vi "_IgnoreInternalData.vi"(8 "error in (no error)":errorcluster, 10 "ignore internal data(T)":bool, 11 "Variant in":variant) -> (0 "error out":errorcluster, 3 "Variant out":variant)   [LabVIEW 2017, in "TagDB(DEV).lvlib"]
uses:
  TagDB(DEV).lvlib
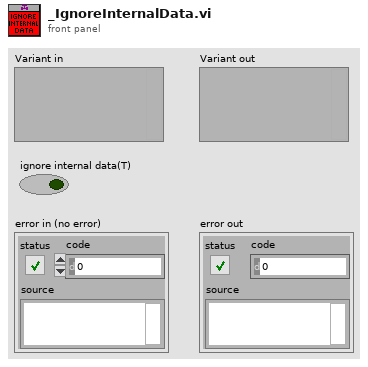
[diagram p1: front panel]
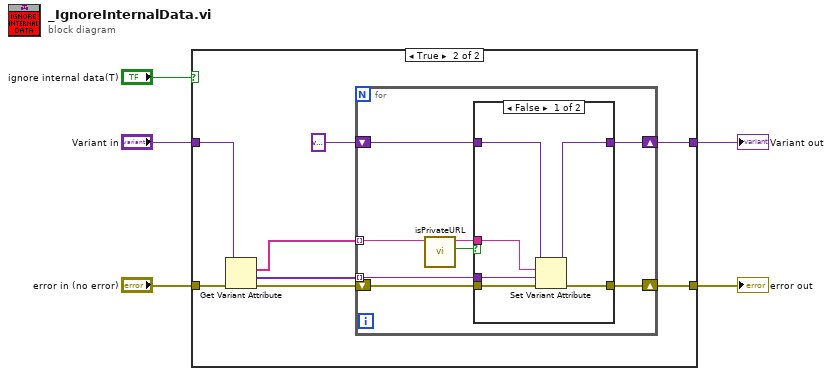
[diagram p0: block diagram]
diagram:
  n1 = case shown="True" "ignore internal data(T)" {
    tunnel: "Variant in" -> [w7 w15]
    tunnel: [w7 w12] -> w3
    tunnel: "error in (no error)" -> [w6 w9]
    tunnel: [w6 w8] -> w5
    frame False {
    }
    frame True {
      n2 = Get Variant Attribute(Variant=w15, error in=w9) -> (names=w14:string[], values=w13:variant[], error out=w10:errorcluster)  [unwired: 2 in, 1 out]
      n3 = for {
        tunnel: w14 -> [w22] mode=indexing
        tunnel: w13 -> [w21] mode=indexing
        shift-right: [w20] -> w12
        shift-left: variant ("Variant") -> [w23]
        shift-right: [w18] -> w8
        shift-left: w10 -> [w19]
        n4 = call "isPrivateURL.vi"("URL"=w22) -> ("private?"=w16:bool, "URL (dup)"=w17:string)  [unwired: 9 in]
        n5 = case shown="False" w16 {
          tunnel: w23 -> [w29 w31]
          tunnel: w17 -> [w28 _]
          tunnel: w21 -> [w27 _]
          tunnel: [w26 w31] -> w20
          tunnel: w19 -> [w25 w30]
          tunnel: [w24 w30] -> w18
          frame False {
            n6 = Set Variant Attribute(Variant=w29, name=w28, value=w27, error in=w25) -> (Variant out=w26:variant, error out=w24:errorcluster)  [unwired: 1 out]
          }
          frame True {
          }
        }
      }
    }
  }
  "error out" <- w5
  "Variant out" <- w3
